vi "Main.vi"(11 "Module Admin":refnum<class "Delacor_lib_QMH_Module Admin.lvclass">) -> ()   [LabVIEW 2026, in "Device Manager.lvlib"]
doc: "This template is based off of the Queued Message Handler design pattern and the Queued Message Handler project template that ships with LabVIEW.\n\nThe main difference is that the queue is private to this module and communication between modules is performed via Broadcast and Request events.\n\nRequest events are wrapped in public API methods and are handled in the Event Handling Loop (EHL) of this VI. Any module can register for Broadcast events sent by this module. The EHL generates messages based on user interface actions.\n\nThe Message Handling Loop (MHL) processes messages generated by the EHL, or by other messages. The messages are string values, so new messages can be added easily to the Message Cases case structure in the MHL. Each message cluster can also provide an optional value for Message Data, which is a variant that can be converted to whatever message-specific data is required.\n_____\nBased on DQMH Dev Tools: Project Template 7.1.2.1547."
uses:
  Device Manager.lvlib
  <vilib>/Delacor/Delacor QMH/Libraries/Module Admin_class/Delacor_lib_QMH_Module Admin.lvclass
  Module Data--cluster.ctl
  Stop Argument--cluster.ctl
  <vilib>/Delacor/Delacor QMH/Libraries/Message Queue_class/Delacor_lib_QMH_Message Queue.lvclass/Delacor_lib_QMH_Message Queue.ctl
  <vilib>/Delacor/Delacor QMH/Libraries/Module Admin_class/Delacor_lib_QMH_Module Admin.lvclass/Delacor_lib_QMH_Module Admin.ctl
  Launch Front Panel (Reply Payload)--cluster.ctl
  Front Panel Emulator/Position Change Requested Argument--cluster.ctl
  Servo Motor Emulator/Temperature Updated Argument--cluster.ctl
  Servo Motor Emulator/Humidity Updated Argument--cluster.ctl
  <vilib>/Utility/miscctls.llb/LVPointTypeDef.ctl
  <vilib>/Delacor/Delacor QMH/Libraries/Message Queue_class/Delacor_lib_QMH_Enqueue Message (Single).vi
  <vilib>/Delacor/Delacor QMH/Libraries/Module Admin_class/Delacor_lib_QMH_Get External Launch.vi
  <vilib>/Delacor/Delacor QMH/Libraries/Message Queue_class/Delacor_lib_QMH_Message Queue.lvclass
  Front Panel Emulator/Front Panel Emulator.lvlib
  Servo Motor Emulator/Servo Motor Emulator.lvlib
panel:
  in  "Show Panel":bool
  in  "Show Motor":bool
  out "error out":errorcluster
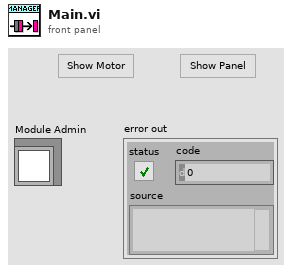
[diagram p1: front panel]
types:
  T1 = typedef "Front Panel Emulator.lvlib/Broadcast Events--cluster.ctl" = cluster{"Module Did Init":refnum<user-event>, "Status Updated":refnum<user-event>, "Error Reported":refnum<user-event>, "Module Did Stop":refnum<user-event>, "Update Module Execution Status":refnum<user-event>, "Position Change Requested":refnum<user-event>}
  T2 = typedef "Servo Motor Emulator.lvlib/Broadcast Events--cluster.ctl" = cluster{"Module Did Init":refnum<user-event>, "Status Updated":refnum<user-event>, "Error Reported":refnum<user-event>, "Module Did Stop":refnum<user-event>, "Update Module Execution Status":refnum<user-event>, "Temperature Updated":refnum<user-event>, "Humidity Updated":refnum<user-event>}
  T3 = typedef "Device Manager.lvlib/Request Events--cluster.ctl" = cluster{"Stop Module":refnum<user-event>, "Show Panel":refnum<user-event>, "Hide Panel":refnum<user-event>, "Get Module Execution Status":refnum<user-event>, "Show Diagram":refnum<user-event>, "Private.Launch Front Panel":refnum<user-event>}
  T4 = typedef "Device Manager.lvlib/Module Data--cluster.ctl" = cluster{"Status":string}
  T5 = enum32{"invalid lock state", "Not Locked", "Locked (No Password)", "Password-protected"}
  T6 = typedef "Device Manager.lvlib/Stop Argument--cluster.ctl" = cluster{"Origin":string, "Exit via Stop Module Req?":bool, "Wait for Module to stop?":bool}
  T7 = typedef "Device Manager.lvlib/Launch Front Panel (Reply Payload)--cluster.ctl" = cluster{"error":errorcluster}
  T8 = typedef "Front Panel Emulator.lvlib/Position Change Requested Argument--cluster.ctl" = cluster{"Position":dbl}
  T9 = typedef "Servo Motor Emulator.lvlib/Temperature Updated Argument--cluster.ctl" = cluster{"Temperature":dbl}
  T10 = typedef "Servo Motor Emulator.lvlib/Humidity Updated Argument--cluster.ctl" = cluster{"Humidity":dbl}
  T11 = typedef "LVPointTypeDef.ctl" = cluster{"Horizontal":i16, "Vertical":i16}
  T12 = enum32{"Invalid", "Standard", "Closed", "Hidden", "Minimized", "Maximized"}
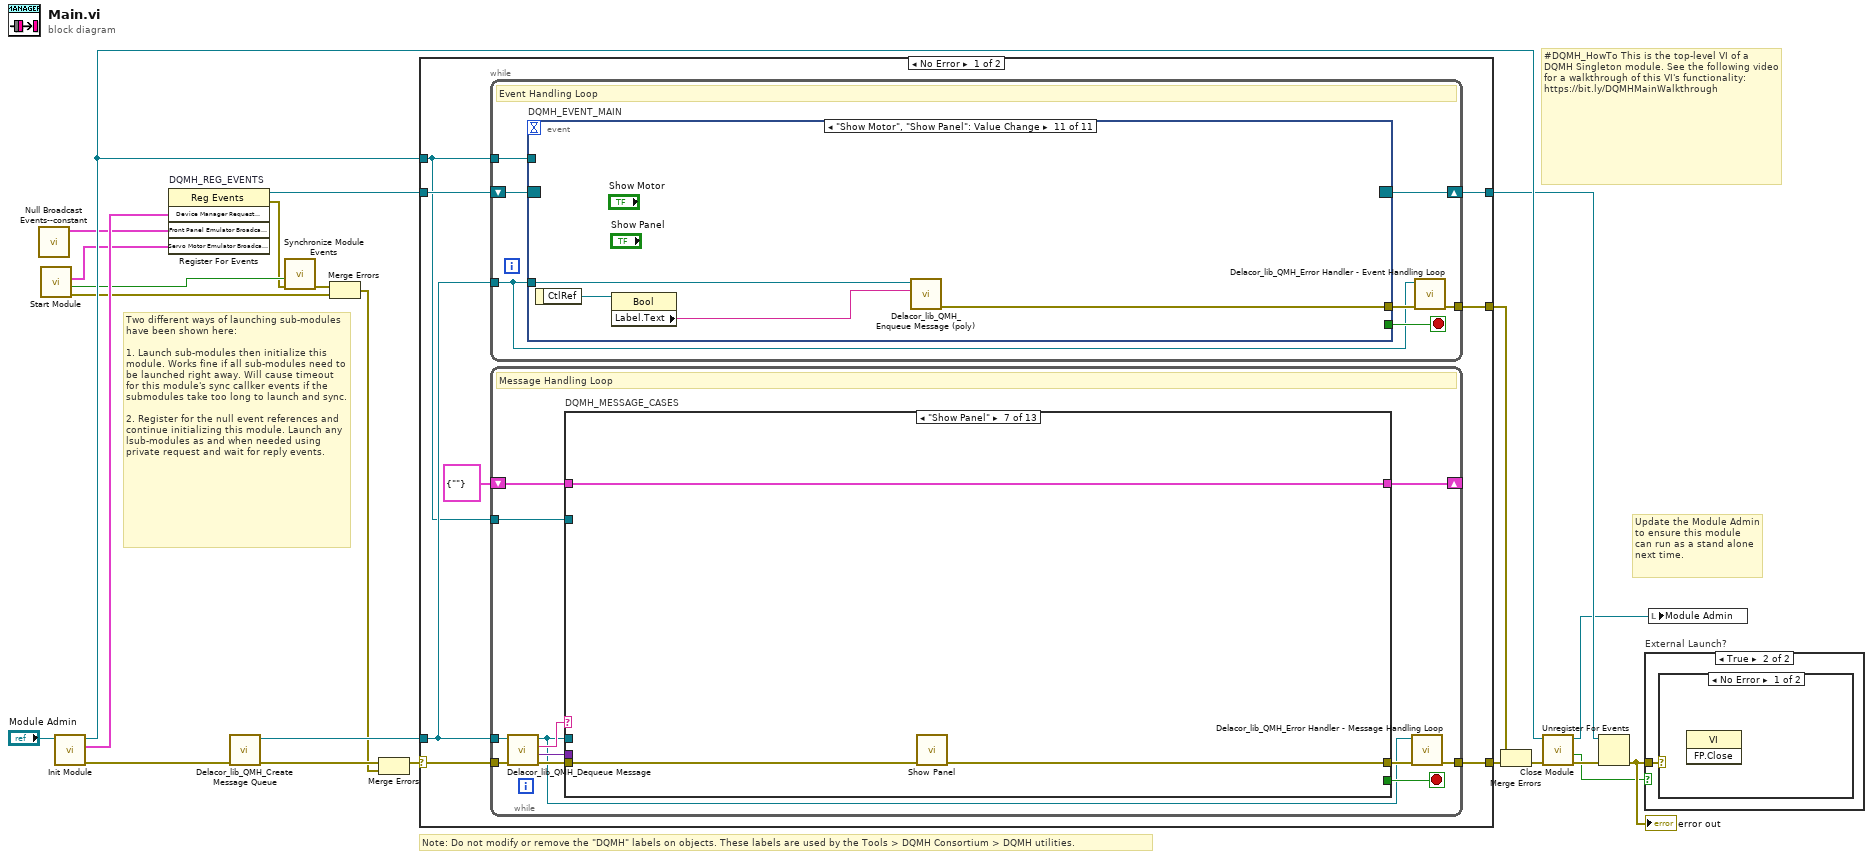
[diagram p0: block diagram]
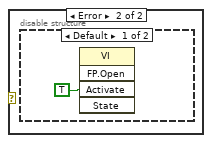
[diagram p3: hidden frame]
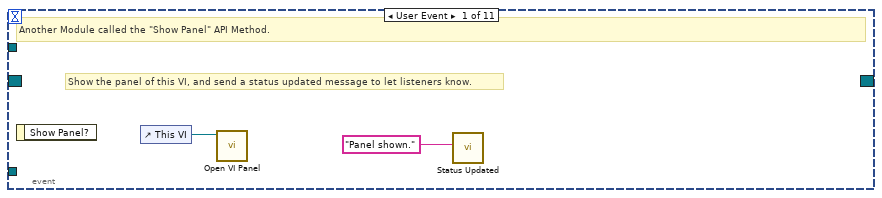
[diagram p5: hidden frame]
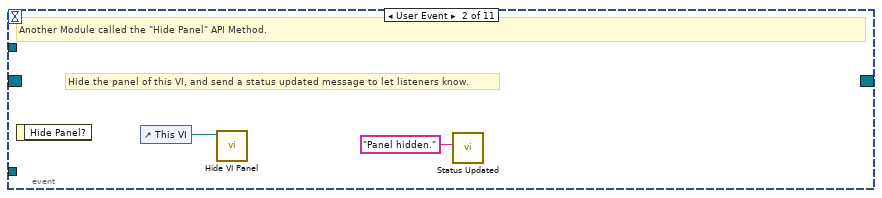
[diagram p6: hidden frame]
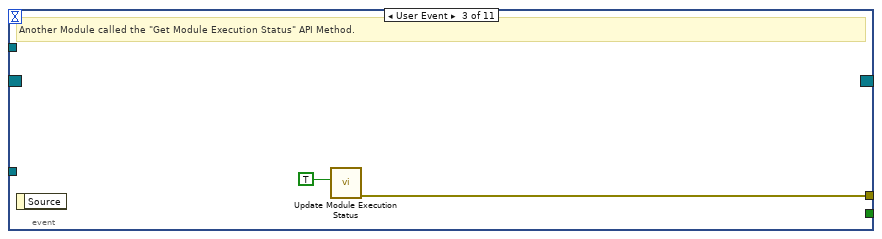
[diagram p7: hidden frame]
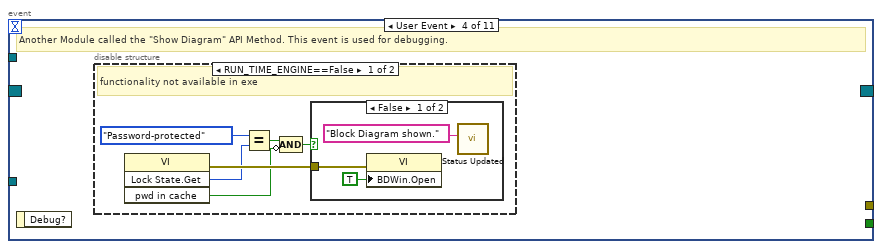
[diagram p8: hidden frame]
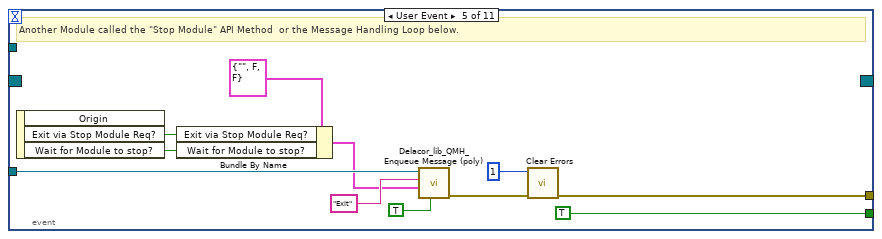
[diagram p11: hidden frame]
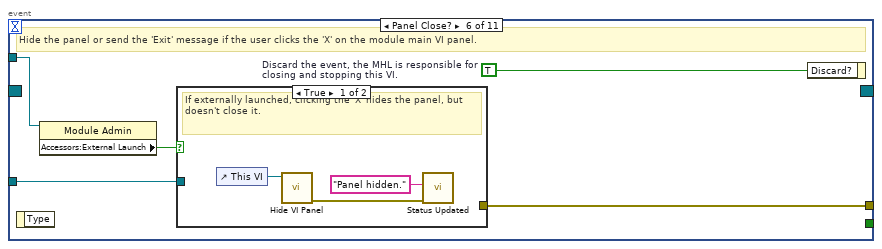
[diagram p12: hidden frame]
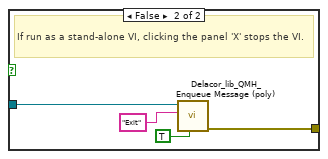
[diagram p13: hidden frame]
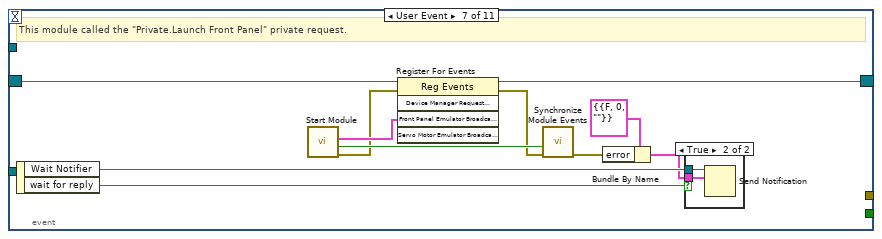
[diagram p14: hidden frame]
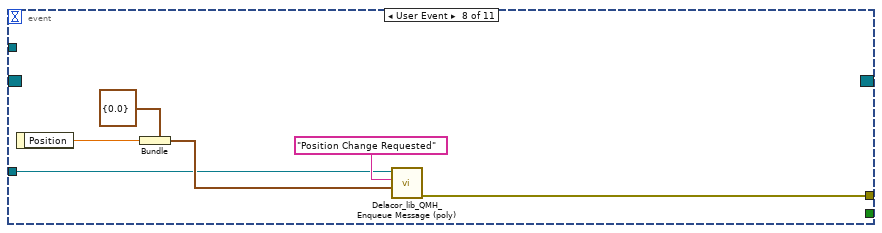
[diagram p16: hidden frame]
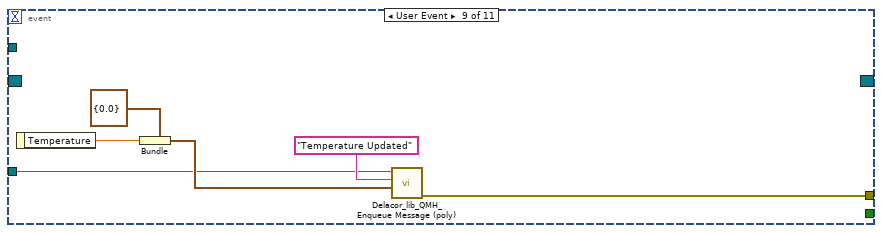
[diagram p17: hidden frame]
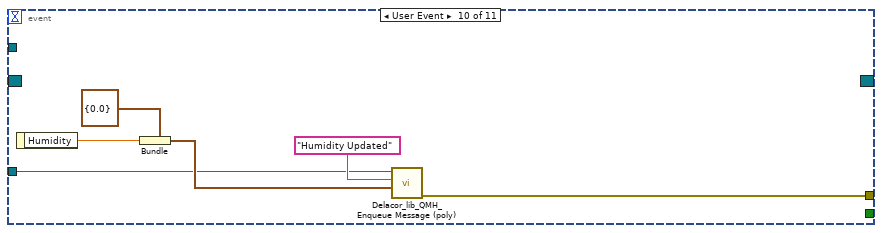
[diagram p18: hidden frame]
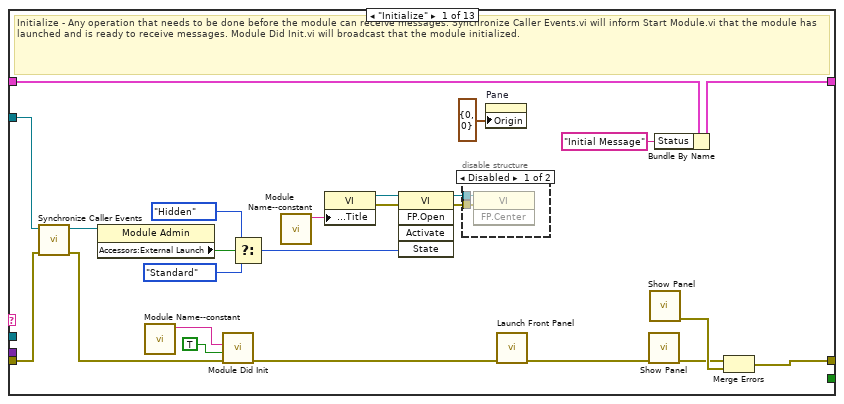
[diagram p19: hidden frame]
diagram:
  # "Two different ways of launching sub-modules have been shown here:\n\n1. Launch sub-modules then initialize this module. Works fine if all sub-modules need to be launched right away. Will cause timeout for this module's sync callker events if the submodules take too long to launch and sync.\n\n2. Register for the null event references and continue initializing this module. Launch any lsub-modules as and when needed using private request and wait for reply events."
  # "#DQMH_HowTo This is the top-level VI of a DQMH Singleton module. See the following video for a walkthrough of this VI's functionality: https://bit.ly/DQMHMainWalkthrough"
  # "Note: Do not modify or remove the \"DQMH\" labels on objects. These labels are used by the Tools > DQMH Consortium > DQMH utilities."
  # "Update the Module Admin to ensure this module can run as a stand alone next time."
  n1 = call "Null Broadcast Events--constant.vi"() -> ("Front Panel Emulator Broadcast Events"=w1:T1)  [unwired: 11 in]
  n2 = call "Start Module.vi"() -> ("error out"=w4:errorcluster, "Wait for Event Sync?"=w6:bool, "Servo Motor Emulator Broadcast Events"=w7:T2)  [unwired: 7 in, 2 out]
  n3 = call "Init Module.vi"("Singleton Module Admin in"="Module Admin") -> ("error out"=w22:errorcluster, "Device Manager Request Events"=w12:T3, "Singleton Module Admin out"=w15:refnum<class "Delacor_lib_QMH_Module Admin.lvclass">)  [unwired: 8 in]
  n4 = register-events "DQMH_REG_EVENTS"(w12, w1, w7) -> (reference out=w13:refnum<event-registration>, error out=w3:errorcluster)  [unwired: 2 in]
  n5 = call <vilib>:"Delacor_lib_QMH_Create Message Queue.vi"("error in"=w22) -> ("error out"=w17:errorcluster, "Message Queue"=w11:refnum<class "Delacor_lib_QMH_Message Queue.lvclass">)  [unwired: 9 in]
  n6 = call "Synchronize Module Events.vi"("error in"=w3, "Wait for Event Sync?"=w6) -> ("error out"=w5:errorcluster)  [unwired: 9 in]
  n7 = Merge Errors(w5, w4) -> (w2:errorcluster)
  n8 = Merge Errors(w17, w2) -> (w16:errorcluster)
  n9 = case shown="No Error" w16 {
    selector: w16 -> [w29 w249]
    tunnel: [w31 w248] -> w23
    tunnel: [w28 w247] -> w14
    tunnel: w13 -> [w26 w247]
    tunnel: w11 -> [w25 w242]
    tunnel: [w30 _] -> w20
    tunnel: w15 -> [w24 w243]
    frame No Error {
      n10 = while {
        tunnel: w25 -> [w32]
        shift-right: [w35] -> w28
        shift-left: w26 -> [w36]
        tunnel: [w37] -> w30
        tunnel: w24 -> [w33]
        stop <- w34 stop-if-true
        # "Event Handling Loop"
        n11 = event "DQMH_EVENT_MAIN" shown="[10] \"Show Motor\", \"Show Panel\": Value Change" {
          selector: w36 -> [_ _ _ _ _ _ w83 _ _ _ _]
          dyn-events: [_ _ _ _ _ _ w82 _ _ _ _] -> w35
          timeout: _ -> [_ _ _ _ _ _ _ _ _ _ _]
          tunnel: [_ _ _ _ TRUE ("Discard?") _ _ _ _ _ _] -> w34
          tunnel: w32 -> [_ _ _ _ w60 w67 _ w91 w97 w103 w111]
          tunnel: [_ _ w44 _ w63 w69 _ w90 w96 w102 w110] -> w38
          tunnel: w33 -> [_ _ _ _ _ w66 _ _ _ _ _]
          event User Event {
            # "Show the panel of this VI, and send a status updated message to let listeners know."
            # "Another Module called the \"Show Panel\" API Method."
            n12 = event-data() -> ()  [unwired: 1 in, 1 out]
            n13 = control-ref of="This VI"() -> (w40:refnum<vi>)
            n14 = call "Open VI Panel.vi"("VI"=w40) -> ()  [unwired: 10 in, 1 out]
            n15 = call "Status Updated.vi"("Status"="Panel shown." ("format string")) -> ()  [unwired: 10 in, 1 out]
          }
          event User Event {
            # "Hide the panel of this VI, and send a status updated message to let listeners know."
            # "Another Module called the \"Hide Panel\" API Method."
            n16 = event-data() -> ()  [unwired: 1 in, 1 out]
            n17 = control-ref of="This VI"() -> (w42:refnum<vi>)
            n18 = call "Hide VI Panel.vi"("VI"=w42) -> ()  [unwired: 10 in, 1 out]
            n19 = call "Status Updated.vi"("Status"="Panel hidden." ("format string")) -> ()  [unwired: 10 in, 1 out]
          }
          event User Event {
            # "Another Module called the \"Get Module Execution Status\" API Method."
            n20 = event-data() -> ()  [unwired: 1 in, 1 out]
            n21 = call "Update Module Execution Status.vi"("Running?"=TRUE) -> ("error out"=w44:errorcluster)  [unwired: 10 in]
          }
          event User Event {
            # "Another Module called the \"Show Diagram\" API Method. This event is used for debugging."
            n22 = event-data() -> ()  [unwired: 1 in, 1 out]
            n23 = disable-structure shown="RUN_TIME_ENGINE==False" {
              frame condition #0 (active) {
                # "functionality not available in exe"
                n24 = invoke on="Invoke Node" class="VI" method="Lock State.Get"() -> (error out=w50:errorcluster, "Get Lock State"=w49:T5, "pwd in cache"=w46:bool)  [unwired: 4 in, 1 out]
                n25 = Equal?(x=T5."Password-protected", y=w49) -> (x = y?=w47:bool)
                n26 = Compound Arithmetic op=AND(w47, invert w46) -> (w45:bool)
                n27 = case shown="False" w45 {
                  tunnel: w50 -> [w53 _]
                  frame False {
                    n28 = property on="Property Node" class="VI"(error in=w53, "BDWin.Open"=TRUE ("Block Diagram Window:Open")) -> ()  [unwired: 1 in, 2 out]
                    n29 = call "Status Updated.vi"("Status"="Block Diagram shown." ("format string")) -> ()  [unwired: 10 in, 1 out]
                  }
                  frame True {
                    # "Password-protected VI, and the password is not in the cache. Do not show the diagram."
                  }
                }
              }
              frame condition #1 {
              }
            }
          }
          event User Event {
            # "Another Module called the \"Stop Module\" API Method  or the Message Handling Loop below."
            n30 = event-data() -> ("Exit via Stop Module Req?"=w56:bool, "Wait for Module to stop?"=w55:bool)  [unwired: 1 in, 1 out]
            n31 = Bundle By Name(cluster=T6 {"Origin"="", "Exit via Stop Module Req?"=FALSE, "Wait for Module to stop?"=FALSE} ("Stop Argument"), "Exit via Stop Module Req?"=w56, "Wait for Module to stop?"=w55) -> (w54:T6)
            n32 = call-poly <vilib>:"Delacor_lib_QMH_Enqueue Message (poly).vi"("Priority Message? (F)"=TRUE, "Message Data"=w54, "Message"="Exit", "Message Queue in"=w60) -> ("error out"=w64:errorcluster)  [unwired: 6 in, 1 out]
            n33 = call <vilib>:"Clear Errors.vi"("error in (no error)"=w64, "specific error code to clear (0: all)"=1) -> ("error out"=w63:errorcluster)  [unwired: 4 in, 1 out]
          }
          event Panel Close? {
            w68 = TRUE  # Discard the event, the MHL is responsible for closing and stopping this VI.
            # "Hide the panel or send the 'Exit' message if the user clicks the 'X' on the module main VI panel."
            n34 = event-data() -> ()  [unwired: 1 in, 1 out]
            n35 = property on="Property Node" class="Module Admin"(reference=w66) -> ("Accessors:External Launch"=w65:bool)  [unwired: 1 in, 2 out]
            n36 = case shown="True" w65 {
              tunnel: w67 -> [_ w75]
              tunnel: [_ w76] -> w69
              frame True {
                # "If externally launched, clicking the 'X' hides the panel, but doesn't close it."
                n37 = control-ref of="This VI"() -> (w72:refnum<vi>)
                n38 = call "Hide VI Panel.vi"("VI"=w72) -> ("error out"=w70:errorcluster)  [unwired: 10 in]
                n39 = call "Status Updated.vi"("error in"=w70, "Status"="Panel hidden." ("format string")) -> ()  [unwired: 9 in, 1 out]
              }
              frame False {
                # "If run as a stand-alone VI, clicking the panel 'X' stops the VI."
                n40 = call-poly <vilib>:"Delacor_lib_QMH_Enqueue Message (poly).vi"("Priority Message? (F)"=TRUE, "Message"="Exit", "Message Queue in"=w75) -> ("error out"=w76:errorcluster)  [unwired: 7 in, 1 out]
              }
            }
            n41 = event-data ("Event Filter Node")("Discard?"=w68) -> ()  [unwired: 1 in, 1 out]
          }
          event User Event {
            # "This module called the \"Private.Launch Front Panel\" private request."
            n42 = event-data() -> ("Wait Notifier"=w87:refnum<notifier>, "wait for reply"=w86:bool)  [unwired: 1 in]
            n43 = call "Start Module.vi"() -> ("error out"=w78:errorcluster, "Wait for Event Sync?"=w80:bool, "Front Panel Emulator Broadcast Events"=w81:T1)  [unwired: 7 in, 2 out]
            n44 = register-events(reference=w83, error in=w78, w81) -> (reference out=w82:refnum<event-registration>, error out=w79:errorcluster)  [unwired: 2 in]
            n45 = call "Synchronize Module Events.vi"("error in"=w79, "Wait for Event Sync?"=w80) -> ("error out"=w77:errorcluster)  [unwired: 9 in]
            n46 = Bundle By Name(cluster=T7 {"error"={"status"=FALSE, "code"=0, "source"=""}} ("Launch Front Panel (Reply Payload)"), "error"=w77) -> (w85:T7)
            n47 = case "DQMH_FIRE_NOTIFIER" shown="True" w86 {
              tunnel: w87 -> [_ w89]
              tunnel: w85 -> [_ w88]
              frame False {
              }
              frame True {
                n48 = Send Notification(notification=w88, notifier=w89) -> ()  [unwired: 1 in, 2 out]
              }
            }
          }
          event User Event {
            n49 = event-data() -> ("Position"=w93:dbl)  [unwired: 1 in]
            n50 = Bundle(cluster=T8 {"Position"=0.0} ("Position Change Requested Argument"), "Position"=w93) -> (w92:T8)
            n51 = call-poly <vilib>:"Delacor_lib_QMH_Enqueue Message (poly).vi"("Message Data"=w92, "Message"="Position Change Requested", "Message Queue in"=w91) -> ("error out"=w90:errorcluster)  [unwired: 7 in, 1 out]
          }
          event User Event {
            n52 = event-data() -> ("Temperature"=w99:dbl)  [unwired: 1 in]
            n53 = Bundle(cluster=T9 {"Temperature"=0.0} ("Temperature Updated Argument"), "Temperature"=w99) -> (w98:T9)
            n54 = call-poly <vilib>:"Delacor_lib_QMH_Enqueue Message (poly).vi"("Message Data"=w98, "Message"="Temperature Updated", "Message Queue in"=w97) -> ("error out"=w96:errorcluster)  [unwired: 7 in, 1 out]
          }
          event User Event {
            n55 = event-data() -> ("Humidity"=w105:dbl)  [unwired: 1 in]
            n56 = Bundle(cluster=T10 {"Humidity"=0.0} ("Humidity Updated Argument"), "Humidity"=w105) -> (w104:T10)
            n57 = call-poly <vilib>:"Delacor_lib_QMH_Enqueue Message (poly).vi"("Message Data"=w104, "Message"="Humidity Updated", "Message Queue in"=w103) -> ("error out"=w102:errorcluster)  [unwired: 7 in, 1 out]
          }
          event "Show Motor", "Show Panel": Value Change {
            n58 = event-data() -> ("CtlRef"=w109:refnum<vi>)  [unwired: 1 in]
            n59 = property class="Bool"(reference=w109) -> ("Label.Text"=w108:string)  [unwired: 1 in, 2 out]
            n60 = call-poly <vilib>:"Delacor_lib_QMH_Enqueue Message (poly).vi"("Message"=w108, "Message Queue in"=w111) -> ("error out"=w110:errorcluster)  [unwired: 8 in, 1 out]
          }
        }
        n61 = call-dynamic "Delacor_lib_QMH_Error Handler - Event Handling Loop.vi"("error in"=w38, "Message Queue in"=w32) -> ("dup error in"=w37:errorcluster)  [unwired: 8 in, 1 out]
      }
      n62 = while {
        tunnel: w25 -> [w112]
        shift-right: [w120] -> _
        shift-left: T4 {"Status"=""} ("Data Cluster") -> [w121]
        tunnel: w29 -> [w123]
        tunnel: [w115] -> w31
        tunnel: w24 -> [w116]
        stop <- w119 stop-if-true
        # "Message Handling Loop"
        n63 = call-dynamic "Delacor_lib_QMH_Dequeue Message.vi"("error in"=w123, "Message Queue in"=w112) -> ("error out"=w122:errorcluster, "Message Data"=w117:variant, "Message"=w118:string, "Message Queue out"=w113:refnum<class "Delacor_lib_QMH_Message Queue.lvclass">)  [unwired: 6 in]
        n64 = case "DQMH_MESSAGE_CASES" shown="\"Show Panel\"" w118 {
          selector: w118 -> [_ _ _ _ _ _ _ _ _ _ _ _ w237]
          tunnel: w113 -> [_ _ _ _ _ _ _ _ _ _ w199 w225 _]
          tunnel: w122 -> [w145 w151 w156 w164 w172 w176 w179 w184 w186 w195 w206 w231 w240]
          tunnel: [w124 w151 w152 w160 w168 w177 w180 w183 w186 w194 w202 w226 w241] -> w114
          tunnel: w121 -> [w135 w150 w159 w167 w175 w178 w181 w182 w185 w192 w201 w224 w238]
          tunnel: [w134 w150 w159 w167 w175 w178 w181 w182 w185 w192 w201 w224 w238] -> w120
          tunnel: [_ _ _ _ _ _ _ _ _ _ _ w223 _] -> w119
          tunnel: w117 -> [_ _ w158 w166 w174 _ _ _ _ _ w200 w222 _]
          tunnel: w116 -> [w136 _ _ _ _ _ _ _ _ _ w198 w217 _]
          frame "Initialize" {
            # "Initialize - Any operation that needs to be done before the module can receive messages. Synchronize Caller Events.vi will inform Start Module.vi that the module has launched and is ready to receive messages. Module Did Init.vi will broadcast that the module initialized."
            n65 = call "Synchronize Caller Events.vi"("error in"=w145, "Singleton Module Admin in"=w136) -> ("error out"=w144:errorcluster, "Singleton Module Admin out"=w131:refnum<class "Delacor_lib_QMH_Module Admin.lvclass">)  [unwired: 8 in]
            n66 = property on="Property Node" class="Module Admin"(reference=w131) -> ("Accessors:External Launch"=w140:bool)  [unwired: 1 in, 2 out]
            n67 = call "Module Name--constant.vi"() -> ("Module Name"=w132:string)  [unwired: 11 in]
            n68 = call "Module Did Init.vi"("error in"=w144, "Initialized?"=TRUE, "Origin"=w132) -> ("error out"=w128:errorcluster)  [unwired: 8 in]
            n69 = Select(t=T12."Hidden" ("State"), s=w140, f=T12."Standard" ("State")) -> (s? t:f=w137:T12)
            n70 = call "Module Name--constant.vi"() -> ("Module Name"=w143:string)  [unwired: 11 in]
            n71 = property on="Property Node" class="VI"("Front Panel.Title"=w143) -> (reference out=w142:refnum<vi>, error out=w147:errorcluster)  [unwired: 2 in]
            n72 = invoke on="Invoke Node" class="VI" method="FP.Open"(reference=w142, error in=w147, "State"=w137) -> (reference out=w141:refnum<vi>, error out=w146:errorcluster)  [unwired: 2 in, 3 out]
            n73 = disable-structure shown="Disabled" {
              disable-tunnel: w146 -> [w149 _]
              disable-tunnel: w141 -> [w148 _]
              frame Disabled {
                n74 = invoke on="Invoke Node" class="VI" method="FP.Center"(reference=w148, error in=w149) -> ()  [unwired: 1 in, 3 out]
              }
              frame Enabled {
              }
            }
            n75 = property on="Pane" class="Pane"("Origin"=T11 {"Horizontal"=0, "Vertical"=0}) -> ()  [unwired: 2 in, 2 out]
            n76 = call "Launch Front Panel.vi"("error in"=w128) -> ("error out"=w127:errorcluster)  [unwired: 9 in, 1 out]
            n77 = call "Show Panel.vi"("error in"=w127) -> ("error out"=w125:errorcluster)  [unwired: 10 in]
            n78 = call "Show Panel.vi"() -> ("error out"=w126:errorcluster)  [unwired: 11 in]
            n79 = Bundle By Name(cluster=w135, "Status"="Initial Message" ("Initial Message")) -> (w134:T4)
            n80 = Merge Errors(w125, w126) -> (w124:errorcluster)
          }
          frame "---Module Specific---" {
            # "Separator -- The following cases handle messages specific to this Module."
          }
          frame "Position Change Requested" {
            n81 = Variant To Data(error in=w156, type=T8 {"Position"=0.0} ("Position Change Requested Argument"), Variant=w158) -> (data=w155:T8, error out=w153:errorcluster)
            n82 = Unbundle By Name(w155) -> ("Position"=w154:dbl)
            n83 = call "Update Position.vi"("error in"=w153, "Position"=w154) -> ("error out"=w152:errorcluster)  [unwired: 9 in]
          }
          frame "Temperature Updated" {
            n84 = Variant To Data(error in=w164, type=T9 {"Temperature"=0.0} ("Temperature Updated Argument"), Variant=w166) -> (data=w163:T9, error out=w161:errorcluster)
            n85 = Unbundle By Name(w163) -> ("Temperature"=w162:dbl)
            n86 = call "Update Temperature.vi"("error in"=w161, "Temperature"=w162) -> ("error out"=w160:errorcluster)  [unwired: 9 in]
          }
          frame "Humidity Updated" {
            n87 = Variant To Data(error in=w172, type=T10 {"Humidity"=0.0} ("Humidity Updated Argument"), Variant=w174) -> (data=w171:T10, error out=w169:errorcluster)
            n88 = Unbundle By Name(w171) -> ("Humidity"=w170:dbl)
            n89 = call "Update Humidity.vi"("error in"=w169, "Relative Humidity"=w170) -> ("error out"=w168:errorcluster)  [unwired: 9 in]
          }
          frame "Show Motor" {
            n90 = call "Show Panel.vi"("error in"=w176) -> ("error out"=w177:errorcluster)  [unwired: 10 in]
          }
          frame "Show Panel" {
            n91 = call "Show Panel.vi"("error in"=w179) -> ("error out"=w180:errorcluster)  [unwired: 10 in]
          }
          frame "---Copy This Frame---" {
            # "Duplicate this frame when creating new messages.  Change this comment in the duplicated frame to describe this message."
            n92 = Merge Errors(w184) -> (w183:errorcluster)
          }
          frame "---Exit and Error Handling---" {
            # "Separator - The following cases handle errors and exit messages."
          }
          frame "Simulate MHL Error" {
            # "#DQMH_HowTo The 'Simulate MHL Error' button  illustrates how the MHL handles errors. This event is instructional in nature and can be removed."
            # "Simulate an error occurring at the MHL"
            n93 = call "Module Name--constant.vi"() -> ("Module Name"=w188:string)  [unwired: 11 in]
            n94 = Format Into String(format string="Simulated error originating at Message Handling Loop in %s", w188) -> (resulting string=w189:string)  [unwired: 2 in, 1 out]
            n95 = call <vilib>:"Error Cluster From Error Code.vi"("show call chain? (False)"=TRUE, "error message (\"\")"=w189, "error code (0)"=5001) -> ("error out"=w193:errorcluster)  [unwired: 6 in]
            n96 = Merge Errors(w195, w193) -> (w194:errorcluster)
          }
          frame "Error" {
            # "#DQMH_CodeRecommended - If the module is running in standalone mode (External Launch = FALSE), this code will pop up an error dialog and call the 'Exit' message if an error occurs. Add more fine-grained error management here."
            # "Error - Check the error message data and respond accordingly. This message is sent by the \"Error Handler\" VIs at the end of each loop in this application."
            n97 = property on="Property Node" class="Module Admin"(reference=w198) -> ("Accessors:External Launch"=w197:bool)  [unwired: 1 in, 2 out]
            n98 = Variant To Data(error in=w206, type=errorcluster {"status"=FALSE, "code"=0, "source"=""} ("error constant"), Variant=w200) -> (data=w196:errorcluster, error out=w204:errorcluster)
            n99 = local write "error out"(w196) -> ()
            n100 = call "Error Reported.vi"("Error"=w196) -> ()  [unwired: 10 in, 1 out]
            n101 = case shown="False" w197 {
              tunnel: [w211 _] -> w203
              tunnel: w199 -> [w209 _]
              tunnel: w196 -> [w210 _]
              frame False {
                n102 = disable-structure shown="Default" {
                  disable-tunnel: w210 -> [w212 _]
                  frame condition #0 (active) {
                    # "If the module is running standalone, then pop up an error dialog and call the \"Exit\" message."
                    n103 = call <vilib>:"Simple Error Handler.vi"("error in (no error)"=w212) -> ()  [unwired: 4 in, 5 out]
                  }
                  frame condition #1 {
                    # "To prevent the Simple Error Handler VI from being loaded (e.g. when deploying to a Real-Time target), add the Conditional Disable Symbol \"DQMH_Disable_SEH\" to your project and set it to TRUE."
                  }
                }
                n104 = call-poly <vilib>:"Delacor_lib_QMH_Enqueue Message (poly).vi"("Priority Message? (F)"=TRUE, "Message"="Exit", "Message Queue in"=w209) -> ("error out"=w211:errorcluster)  [unwired: 7 in, 1 out]
              }
              frame True {
                # "If the module was launched externally, calling the Error Reported broadcast VI is the only action performed by the \"Error\" message. The module's caller can then process the error appropriately."
              }
            }
            n105 = Merge Errors(w204, w203) -> (w202:errorcluster)
          }
          frame "Exit" {
            w215 = TRUE  # Wait for Module to Stop
            w216 = 10.0  # Timeout (s)
            w221 = 91  # 91: not all Exit messages will have an argument
            w223 = TRUE  # Stop the VI
            # "Release the message queue reference"
            # "Exit - Exit the application."
            n106 = Variant To Data(error in=w231, type=T6 {"Origin"="", "Exit via Stop Module Req?"=FALSE, "Wait for Module to stop?"=FALSE} ("Stop Argument"), Variant=w222) -> (data=w219:T6, error out=w228:errorcluster)
            n107 = control-ref of="This VI"() -> (w218:refnum<vi>)
            n108 = call <vilib>:"Clear Errors.vi"("error in (no error)"=w228, "specific error code to clear (0: all)"=w221) -> ("error out"=w230:errorcluster)  [unwired: 4 in, 1 out]
            n109 = call "Handle Exit.vi"("Stop Argument"=w219, "Admin in"=w217, "VI reference"=w218) -> ("error out"=w227:errorcluster)  [unwired: 7 in, 1 out]
            n110 = call-dynamic "Delacor_lib_QMH_Release Message Queue.vi"("error in"=w230, "Message Queue"=w225) -> ("error out"=w229:errorcluster)  [unwired: 9 in]
            n111 = call "Stop Module.vi"("Timeout to Wait for Stop (s) (-1: no timeout)"=w216, "Wait for Module to Stop? (F)"=w215) -> ("error out"=w213:errorcluster)  [unwired: 9 in]
            n112 = call "Stop Module.vi"("Timeout to Wait for Stop (s) (-1: no timeout)"=w216, "Wait for Module to Stop? (F)"=w215) -> ("error out"=w214:errorcluster)  [unwired: 9 in]
            n113 = Merge Errors(w229, w227, w213, w214) -> (w226:errorcluster)
            n114 = call "Error Reported.vi"("Error"=w226) -> ()  [unwired: 10 in, 1 out]
          }
          frame Default {
            # "'Default' case only runs if there is a message that isn't defined in any of the other cases.  Output a programming error."
            n115 = call "Module Name--constant.vi"() -> ("Module Name"=w236:string)  [unwired: 11 in]
            n116 = Format Into String(format string="The invalid message string \"%s\" was received in the Message Handling Loop for module \"%s\".", w237, w236) -> (resulting string=w232:string)  [unwired: 2 in, 1 out]
            n117 = call <vilib>:"Error Cluster From Error Code.vi"("show call chain? (False)"=TRUE, "error message (\"\")"=w232, "error code (0)"=1) -> ("error out"=w239:errorcluster)  [unwired: 6 in]
            n118 = Merge Errors(w240, w239) -> (w241:errorcluster)
          }
        }
        n119 = call-dynamic "Delacor_lib_QMH_Error Handler - Message Handling Loop.vi"("error in"=w114, "Message Queue in"=w113) -> ("dup error in"=w115:errorcluster)  [unwired: 8 in, 1 out]
      }
    }
    frame Error {
      # "Synchronize Caller Events.vi will inform Start Module.vi that the module has launched and will let the code calling Start Module.vi register for broadcasts and would permit the caller receive the broadcast that an error occurred at launch time."
      n120 = call-dynamic "Delacor_lib_QMH_Release Message Queue.vi"("error in"=w249, "Message Queue"=w242) -> ("error out"=w248:errorcluster)  [unwired: 9 in]
      n121 = call "Synchronize Caller Events.vi"("Singleton Module Admin in"=w243) -> ("error out"=w250:errorcluster)  [unwired: 9 in, 1 out]
      n122 = call "Module Name--constant.vi"() -> ("Module Name"=w246:string)  [unwired: 11 in]
      n123 = Format Into String(format string="An error occurred during initialization. %s is no longer running.", w246) -> (resulting string=w244:string)  [unwired: 2 in, 1 out]
      n124 = Merge Errors(w248, w250) -> (w251:errorcluster)
      n125 = call "Error Reported.vi"("Additional Information"=w244, "Error"=w251) -> ()  [unwired: 9 in, 1 out]
    }
  }
  n126 = Merge Errors(w20, w23) -> (w19:errorcluster)
  n127 = call "Close Module.vi"("error in"=w19, "Module Admin in"=w15) -> ("error out"=w21:errorcluster, "External Launch"=w8:bool, "Module Admin out"=w9:refnum<class "Delacor_lib_QMH_Module Admin.lvclass">)  [unwired: 7 in]
  n128 = Unregister For Events(event registration refnum=w14, error in=w21) -> (error out=w18:errorcluster)
  "error out" <- w18
  n129 = case "External Launch?" shown="True" w8 {
    tunnel: w18 -> [_ w252]
    frame False {
    }
    frame True {
      n130 = case shown="No Error" w252 {
        frame No Error {
          n131 = invoke on="Invoke Node" class="VI" method="FP.Close"() -> ()  [unwired: 3 in, 3 out]
        }
        frame Error {
          n132 = disable-structure shown="Default" {
            frame condition #0 (active) {
              n133 = invoke class="VI" method="FP.Open"("Activate"=TRUE ("Activate?")) -> ()  [unwired: 4 in, 5 out]
            }
            frame condition #1 {
              # "Don't show panel on error if running inside a built EXE."
            }
          }
        }
      }
    }
  }
  n134 = local write "Module Admin"(w9) -> ()
